vi "Digital IO.vi"() -> ()   [LabVIEW 2011]
panel:
  in  "stop":bool
  out "Din1 31":bool
  out "Din1 30":bool
  out "Din1 29":bool
  out "Din1 28":bool
  out "Din1 27":bool
  out "Din1 26":bool
  out "Din1 25":bool
  out "Din1 24":bool
  out "Din1 23":bool
  out "Din1 22":bool
  out "Din1 21":bool
  out "Din1 20":bool
  out "Din1 19":bool
  out "Din1 18":bool
  out "Din1 17":bool
  out "Din1 16":bool
  out "Din1 15":bool
  out "Din1 14":bool
  out "Din1 13":bool
  out "Din1 12":bool
  out "Din1 11":bool
  out "Din1 10":bool
  out "Din1 9":bool
  out "Din1 8":bool
  out "Din1 7":bool
  out "Din1 6":bool
  out "Din1 5":bool
  out "Din1 4":bool
  out "Din1 3":bool
  out "Din1 2":bool
  out "Din1 1":bool
  out "Din1 0":bool
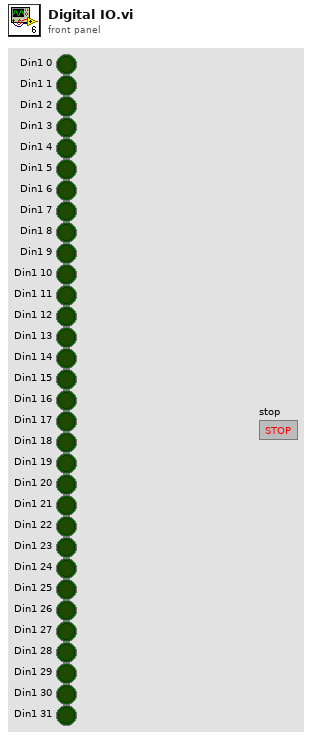
[diagram p1: front panel]
types:
  T1 = enum16{"NC1", "NC2", "Dnet1", "Dnet2", "Dnet3", "Ain1", "Ain2", "Aout1", "Din1", "Din2", "Dout1"}
  T2 = cluster{"Boolean array[0]":bool, "Boolean array[1]":bool, "Boolean array[2]":bool, "Boolean array[3]":bool, "Boolean array[4]":bool, "Boolean array[5]":bool, "Boolean array[6]":bool, "Boolean array[7]":bool, "Boolean array[8]":bool, "Boolean array[9]":bool, "Boolean array[10]":bool, "Boolean array[11]":bool, "Boolean array[12]":bool, "Boolean array[13]":bool, "Boolean array[14]":bool, "Boolean array[15]":bool, "Boolean array[16]":bool, "Boolean array[17]":bool, "Boolean array[18]":bool, "Boolean array[19]":bool, "Boolean array[20]":bool, "Boolean array[21]":bool, "Boolean array[22]":bool, "Boolean array[23]":bool, "Boolean array[24]":bool, "Boolean array[25]":bool, "Boolean array[26]":bool, "Boolean array[27]":bool, "Boolean array[28]":bool, "Boolean array[29]":bool, "Boolean array[30]":bool, "Boolean array[31]":bool}
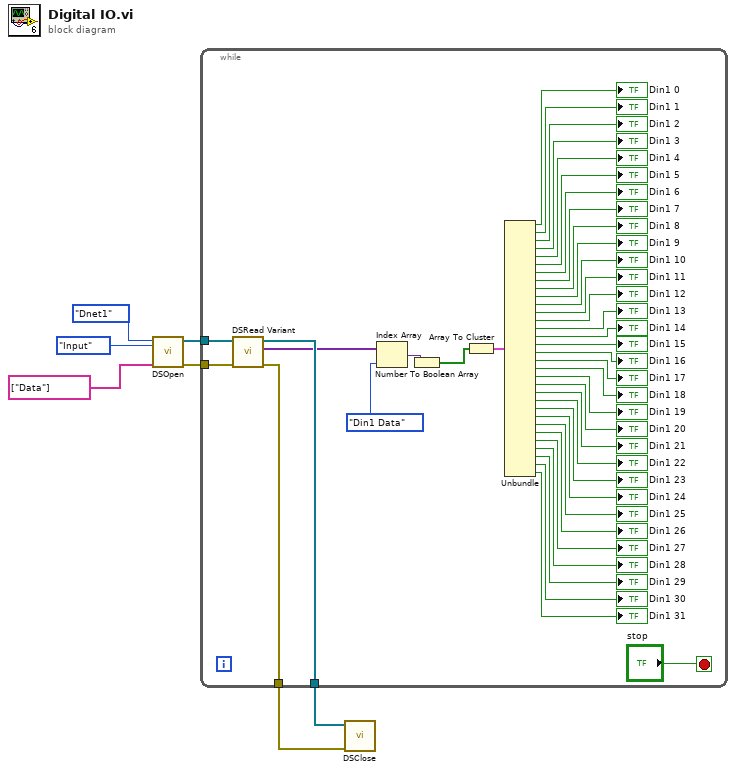
[diagram p0: block diagram]
diagram:
  n1 = call "DSOpen.vi"("Array"=string[] ["Data"], "I/O"=enum16{"Input", "Output"}."Input", "Slot"=T1."Dnet1") -> ("error Out"=w3:errorcluster[], "connection out"=w4:refnum<k13>[])  [unwired: 7 in]
  n2 = while {
    tunnel: w4 -> [w15]
    tunnel: w3 -> [w14]
    tunnel: [w13] -> w2
    tunnel: [w12] -> w1
    stop <- "stop" stop-if-true
    n3 = call "DSRead Variant.vi"("error in"=w14, "connection in"=w15) -> ("error out"=w13:errorcluster[], "data"=w11:variant[], "connection out"=w12:refnum<k13>[])  [unwired: 7 in]
    n4 = Index Array(array=w11, index=enum16{"Din1 Data"}."Din1 Data") -> (element=w9:variant)
    n5 = Number To Boolean Array(number=w9) -> (Boolean array=w8:bool[])
    n6 = Array To Cluster(array=w8) -> (cluster=w49:T2)
    n7 = Unbundle(w49) -> ("Boolean array[0]"=→"Din1 0":bool, "Boolean array[1]"=→"Din1 1":bool, "Boolean array[2]"=→"Din1 2":bool, "Boolean array[3]"=→"Din1 3":bool, "Boolean array[4]"=→"Din1 4":bool, "Boolean array[5]"=→"Din1 5":bool, "Boolean array[6]"=→"Din1 6":bool, "Boolean array[7]"=→"Din1 7":bool, "Boolean array[8]"=→"Din1 8":bool, "Boolean array[9]"=→"Din1 9":bool, "Boolean array[10]"=→"Din1 10":bool, "Boolean array[11]"=→"Din1 11":bool, "Boolean array[12]"=→"Din1 12":bool, "Boolean array[13]"=→"Din1 13":bool, "Boolean array[14]"=→"Din1 14":bool, "Boolean array[15]"=→"Din1 15":bool, "Boolean array[16]"=→"Din1 16":bool, "Boolean array[17]"=→"Din1 17":bool, "Boolean array[18]"=→"Din1 18":bool, "Boolean array[19]"=→"Din1 19":bool, "Boolean array[20]"=→"Din1 20":bool, "Boolean array[21]"=→"Din1 21":bool, "Boolean array[22]"=→"Din1 22":bool, "Boolean array[23]"=→"Din1 23":bool, "Boolean array[24]"=→"Din1 24":bool, "Boolean array[25]"=→"Din1 25":bool, "Boolean array[26]"=→"Din1 26":bool, "Boolean array[27]"=→"Din1 27":bool, "Boolean array[28]"=→"Din1 28":bool, "Boolean array[29]"=→"Din1 29":bool, "Boolean array[30]"=→"Din1 30":bool, "Boolean array[31]"=→"Din1 31":bool)
  }
  n8 = call "DSClose.vi"("error in (no error)"=w2, "connection id"=w1) -> ()  [unwired: 10 in]
